vi "DROPBEAR_Model_Updating_Setter.vi"(8 "error in (no error)":errorcluster, 11 "DROPBEAR_Model_Updating in":refnum<class "DROPBEAR_Model_Updating.lvclass">) -> (0 "error out":errorcluster, 3 "DROPBEAR_Model_Updating out":refnum<class "DROPBEAR_Model_Updating.lvclass">)   [LabVIEW 2021]
uses:
  FEA_Model/FEA_Model.lvclass
  DROPBEAR_Model_Updating.lvclass
  MOCKBEAR/MOCKBEAR.lvclass
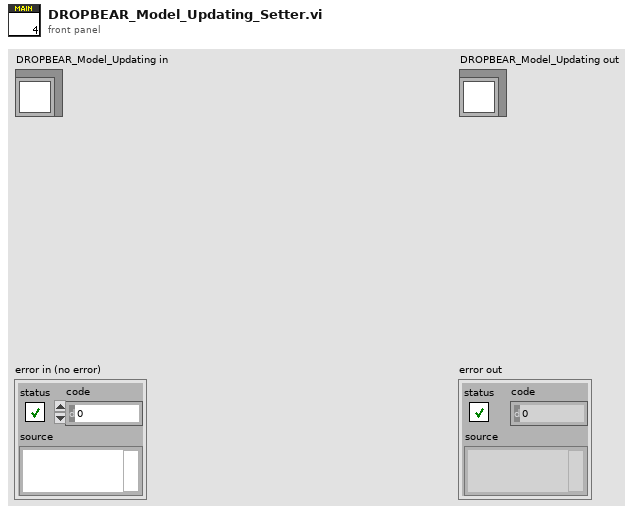
[diagram p1: front panel]
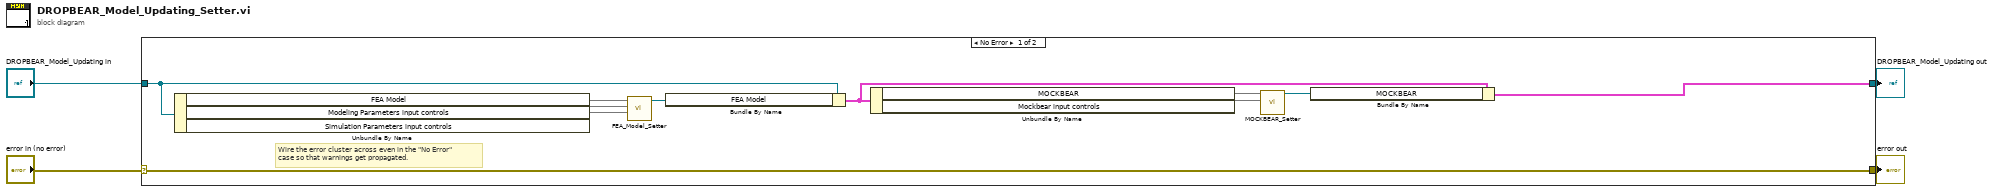
[diagram p0: block diagram]
diagram:
  n1 = case shown="No Error" "error in (no error)" {
    selector: "error in (no error)" -> [w15 w17]
    tunnel: [w15 w17] -> w3
    tunnel: [w14 w16] -> w1
    tunnel: "DROPBEAR_Model_Updating in" -> [w5 w16]
    frame No Error {
      # "Wire the error cluster across even in the \"No Error\"\ncase so that warnings get propagated."
      n2 = Unbundle By Name(w5) -> ("FEA Model"=w13, "Modeling Parameters input controls"=w12, "Simulation Parameters input controls"=w11)
      n3 = call-dynamic "FEA_Model_Setter.vi"("Simulation Parameters input controls"=w11, "Modeling Parameters input controls"=w12, "FEA_Model in"=w13) -> ("FEA_Model out"=w10:refnum<class "FEA_Model.lvclass">)  [unwired: 7 in, 1 out]
      n4 = Bundle By Name(cluster=w5, "FEA Model"=w10) -> (w9:cluster{})
      n5 = Unbundle By Name(w9) -> ("MOCKBEAR"=w8, "Mockbear input controls"=w7)
      n6 = call-dynamic "MOCKBEAR_Setter.vi"("Mockbear input controls"=w7, "MOCKBEAR in"=w8) -> ("MOCKBEAR out"=w6:refnum<class "MOCKBEAR.lvclass">)  [unwired: 8 in, 1 out]
      n7 = Bundle By Name(cluster=w9, "MOCKBEAR"=w6) -> (w14:cluster{})
    }
    frame Error {
    }
  }
  "error out" <- w3
  "DROPBEAR_Model_Updating out" <- w1
